vi "Shared Binary Version (Feature Detection).vi"(8 "error in (no error)":errorcluster) -> (0 "error out":errorcluster, 3 "Version":string)   [LabVIEW 2020, in "feature_detection.lvlib"]
doc: "Get the version of the shared binary file for this component."
uses:
  feature_detection.lvlib
  common/common.lvlib
  common/bin/gartoolkit_fd_32-1.dll
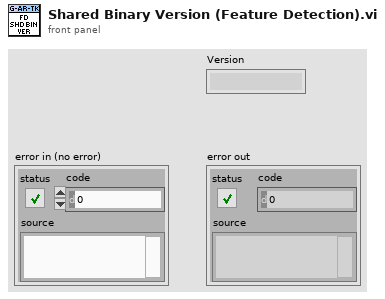
[diagram p1: front panel]
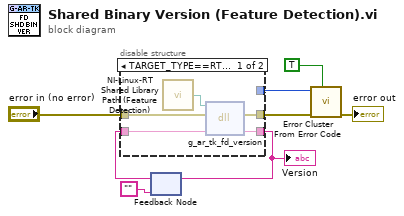
[diagram p0: block diagram]
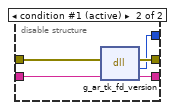
[diagram p2: hidden frame]
diagram:
  n1 = feedback #1("" ("Array")) -> (w3:string)
  n2 = disable-structure shown="TARGET_TYPE==RT&&OS==Linux" {
    disable-tunnel: "error in (no error)" -> [w13 w18]
    disable-tunnel: w3 -> [w11 w17]
    disable-tunnel: [w12 w16] -> w6
    disable-tunnel: [_ w15] -> w5
    disable-tunnel: [w10 w14] -> w4
    frame condition #0 {
      n3 = call "NI-Linux-RT Shared Library Path (Feature Detection).vi"() -> ("Path"=w9:path)
      n4 = dll-call lib="?" fn="g_ar_tk_fd_version" ("g_ar_toolkit.*.*:g_ar_tk_image_draw_line")(path in=w9, error in=w13, "version"=w11) -> (error out=w12:errorcluster, "version"=w10:string)  [unwired: 2 in, 1 out]
    }
    frame condition #1 (active) {
      n5 = dll-call lib="C:/serenial/lib/g-augmented-reality-toolkit/LabVIEW/common/bin/gartoolkit_fd_*-1.*" fn="g_ar_tk_fd_version" ("g_ar_toolkit.*.*:g_ar_tk_image_draw_line")(error in=w18, "version"=w17) -> (error out=w16:errorcluster, "return type"=w15:i32, "version"=w14:string)  [unwired: 2 in, 1 out]
    }
  }
  "Version" <- w4
  n6 = feedback-in #1(w4) -> ()
  n7 = call <vilib>:"Error Cluster From Error Code.vi"("show call chain? (False)"=TRUE, "error in (no error)"=w6, "error code (0)"=w5) -> ("error out"=→"error out":errorcluster)  [unwired: 6 in]
